vi "Write Value2.vi"(10 "Value2":dbl, 11 "Effect Interface in":refnum<class "Effect Interface.lvclass">) -> (3 "Effect Interface out":refnum<class "Effect Interface.lvclass">)   [LabVIEW 2019, in "Effect Interface.lvlib" / "Effect Interface.lvclass"]
uses:
  Effect Interface.lvclass
  Effect Interface.lvclass/Effect Interface.ctl
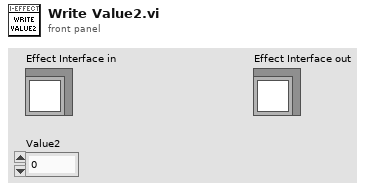
[diagram p1: front panel]
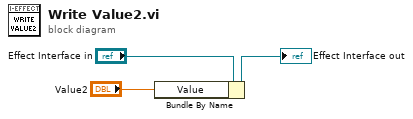
[diagram p0: block diagram]
diagram:
  n1 = Bundle By Name(cluster="Effect Interface in", "Value"="Value2") -> (→"Effect Interface out":refnum<class "Effect Interface.lvclass">)
